vi "Start.vi"(8 "error in (no error)":errorcluster, 11 "Process In":refnum<class "Process.lvclass">) -> (0 "error out":errorcluster, 3 "Process Out":refnum<class "Process.lvclass">)   [LabVIEW 2020, in "Process.lvclass"]
doc: "This methods starts the process which runs asyncronously."
uses:
  Process.lvclass
  Process.lvclass/Process.ctl
  Private/SubVIs/Process Launcher.vi
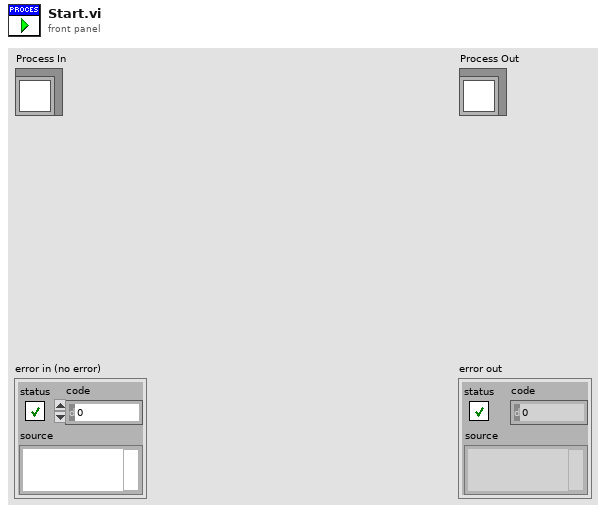
[diagram p1: front panel]
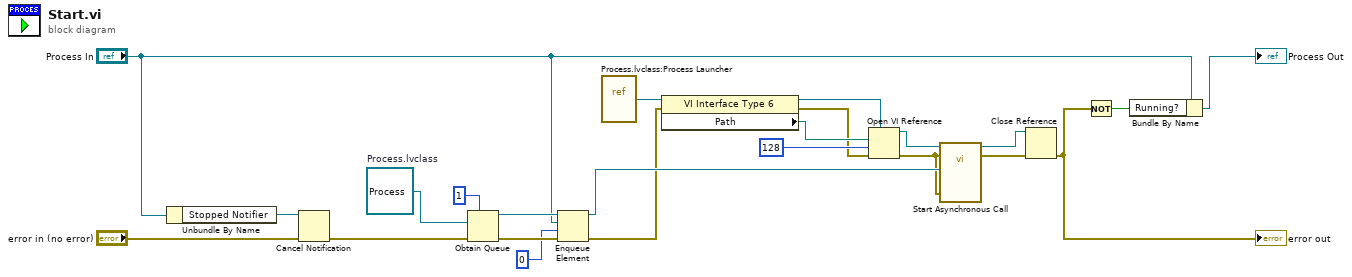
[diagram p0: block diagram]
diagram:
  w20 = refnum<class "Process.lvclass"> refnum  # Process.lvclass
  n1 = Unbundle By Name("Process In") -> ("Stopped Notifier"=w4:refnum<notifier>)
  n2 = Cancel Notification(0:w4, 3:"error in (no error)") -> (11:w2:errorcluster)  [unwired: 2 out]
  n3 = Obtain Queue(max queue size (-1, unlimited)=1, element data type=w20, error in (no error)=w2) -> (queue out=w19:refnum<queue>, error out=w18:errorcluster)  [unwired: 2 in, 1 out]
  n4 = Enqueue Element(queue=w19, element="Process In", timeout in ms (-1)=0, error in (no error)=w18) -> (queue out=w17:refnum<queue>, error out=w11:errorcluster)  [unwired: 1 out]
  n5 = vi-ref "Process.lvclass:Process Launcher.vi"() -> (w16:refnum<vi>)
  n6 = property class="VI Interface Type 6"(reference=w16, error in=w11) -> (reference out=w13:refnum<vi>, error out=w10:errorcluster, "Path"=w12:path)
  n7 = Open VI Reference(type specifier VI Refnum (for type only)=w13, vi path=w12, options=128, error in (no error)=w10) -> (vi reference=w14:refnum<vi>, error out=w9:errorcluster)  [unwired: 2 in]
  n8 = call-by-ref "Start Asynchronous Call"(reference=w14, error in=w9, 8:"error in (no error)"=w9, "Application Queue ref"=w17) -> (reference out=w23:refnum<vi>, error out=w22:errorcluster)  [unwired: 9 in, 1 out]
  n9 = Close Reference(reference=w23, error in (no error)=w22) -> (error out=w7:errorcluster)
  "error out" <- w7
  n10 = Not(x=w7) -> (.not. x?=w6:bool)
  n11 = Bundle By Name(cluster="Process In", "Running?"=w6) -> (→"Process Out":refnum<class "Process.lvclass">)
